vi "ConnectionHandler.vi"(6 "WebSocket Headers":variant, 8 "error in (no error)":errorcluster, 9 "Remote Address":string, 10 "connection ID":refnum<k5>, 11 "References In":variant) -> (0 "error out":errorcluster)   [LabVIEW 2013, in "Connection Handler.lvlib"]
uses:
  Connection Handler.lvlib
  ctl_ClientState.ctl
  <vilib>/Intelligent Energy/Message Queue Helper/ctl_QMH_Message_Typedef.ctl
  ctl_Message.ctl
  <vilib>/Intelligent Energy/Message Queue Helper/MessageQueueHelper.lvlib
  <vilib>/Intelligent Energy/WebSockets API/WebSockets/WebSockets.lvlib
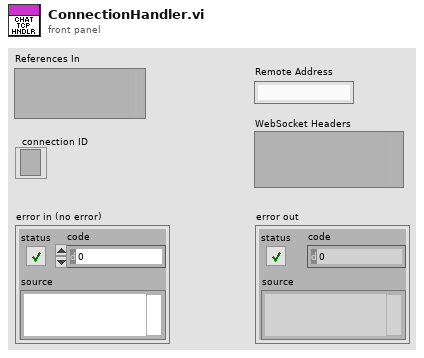
[diagram p1: front panel]
types:
  T1 = typedef "Connection Handler.lvlib/ctl_ClientState.ctl" = cluster{"Conn Ref":refnum<k5>, "IP Address":string, "Hostname":string, "User":cluster{"Username":string, "Read":bool, "Write":bool}}
  T2 = typedef "Connection Handler.lvlib/ctl_Message.ctl" = cluster{"username":string, "message":string}
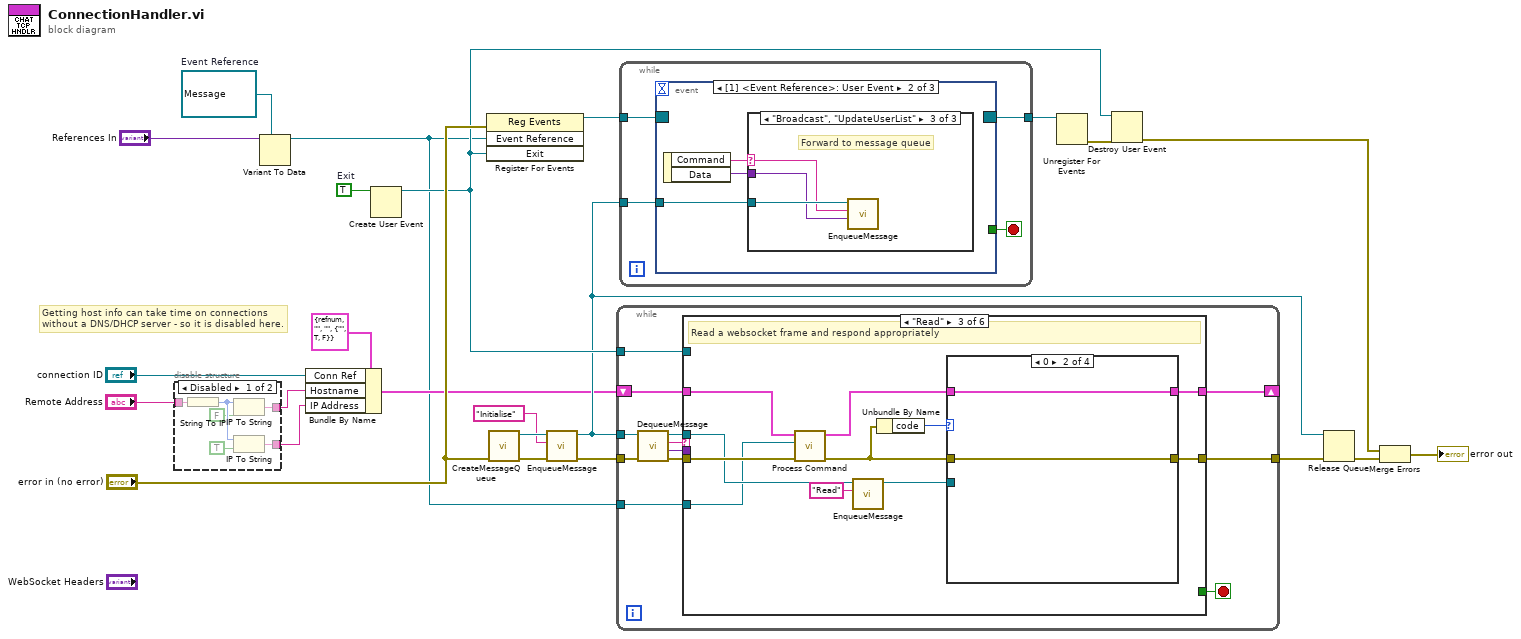
[diagram p0: block diagram]
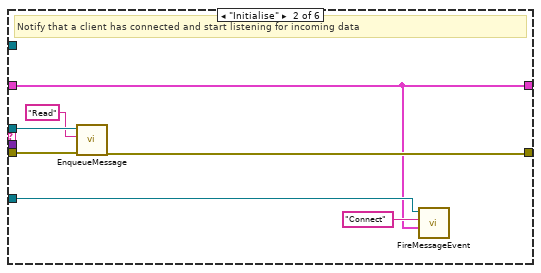
[diagram p4: hidden frame]
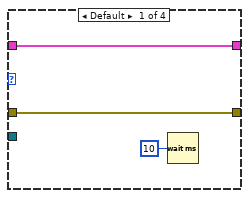
[diagram p5: hidden frame]
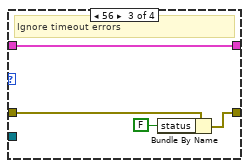
[diagram p6: hidden frame]
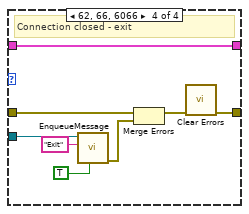
[diagram p7: hidden frame]
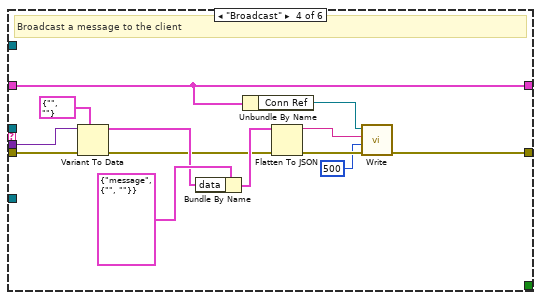
[diagram p8: hidden frame]
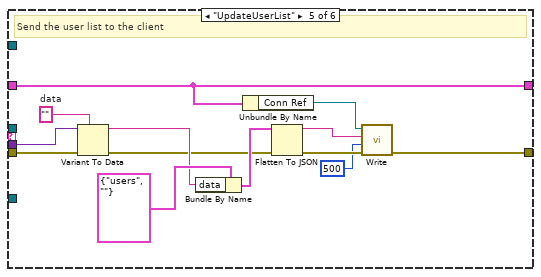
[diagram p9: hidden frame]
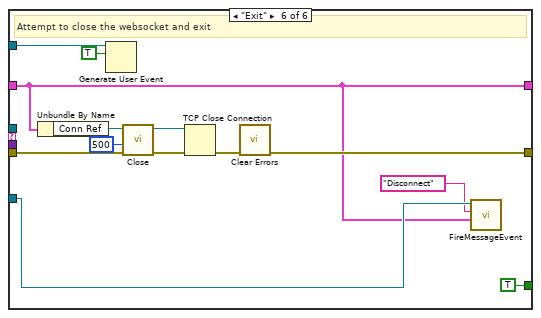
[diagram p10: hidden frame]
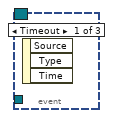
[diagram p11: hidden frame]
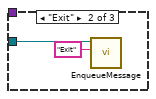
[diagram p13: hidden frame]
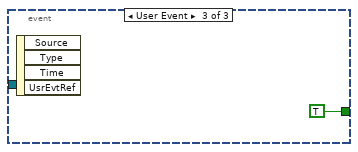
[diagram p14: hidden frame]
diagram:
  w2 = refnum<user-event> refnum  # Event Reference
  w18 = TRUE  # Exit
  # "Getting host info can take time on connections\nwithout a DNS/DHCP server - so it is disabled here."
  n1 = disable-structure shown="Disabled" {
    disable-tunnel: "Remote Address" -> [w27 w31]
    disable-tunnel: [w26 w31] -> w6
    disable-tunnel: [w25 w31] -> w5
    frame Disabled {
      n2 = String To IP(1:w27) -> (0:w30:u32)
      n3 = IP To String(1:FALSE ("dot notation? (F)"), 2:w30) -> (0:w25:string)
      n4 = IP To String(1:TRUE ("dot notation? (F)"), 2:w30) -> (0:w26:string)
    }
    frame Enabled {
    }
  }
  n5 = Variant To Data(type=w2, Variant="References In") -> (data=w1:refnum<user-event>)  [unwired: 1 in, 1 out]
  n6 = Bundle By Name(cluster=T1 {"Conn Ref"=refnum, "IP Address"="", "Hostname"="", "User"={"Username"="", "Read"=TRUE, "Write"=FALSE}} ("State out"), "Conn Ref"="connection ID", "Hostname"=w5, "IP Address"=w6) -> (w4:T1)
  n7 = Create User Event(user event datatype=w18) -> (user event=w15:refnum<user-event>)  [unwired: 1 in, 1 out]
  n8 = register-events(error in="error in (no error)", w1, w15) -> (reference out=w24:refnum<event-registration>)  [unwired: 1 in, 1 out]
  n9 = call <vilib>:"CreateMessageQueue.vi"("error in (no error)"="error in (no error)") -> ("error out"=w14:errorcluster, "queue out"=w11:refnum<queue>)  [unwired: 8 in, 1 out]
  n10 = call <vilib>:"EnqueueMessage.vi"("error in (no error)"=w14, "Message"="Initialise", "queue in"=w11) -> ("error out"=w13:errorcluster, "queue out"=w12:refnum<queue>)  [unwired: 7 in]
  n11 = while {
    tunnel: w12 -> [w43]
    tunnel: w13 -> [w42]
    tunnel: [w33] -> w22
    shift-right: [w36] -> _
    shift-left: w4 -> [w35]
    tunnel: w15 -> [w34]
    tunnel: w1 -> [w32]
    stop <- w37 stop-if-true
    n12 = call <vilib>:"DequeueMessage.vi"("error in (no error)"=w42, "queue in"=w43) -> ("error out"=w40:errorcluster, "Data"=w38:variant, "Command"=w41:string, "queue out"=w39:refnum<queue>)  [unwired: 6 in]
    n13 = case shown="\"Read\"" w41 {
      tunnel: w40 -> [w45 w52 w63 w90 w103 w115]
      tunnel: [w45 w49 w60 w92 w105 w110] -> w33
      tunnel: w39 -> [_ w51 w59 _ _ _]
      tunnel: w38 -> [_ _ _ w89 w102 _]
      tunnel: [_ _ _ _ _ TRUE] -> w37
      tunnel: [w44 w46 w56 w93 w106 w107] -> w36
      tunnel: w35 -> [w44 w46 w54 w93 w106 w107]
      tunnel: w34 -> [_ _ _ _ _ w117]
      tunnel: w32 -> [_ w47 w53 _ _ w109]
      frame Default {
      }
      frame "Initialise" {
        # "Notify that a client has connected and start listening for incoming data"
        n14 = call <vilib>:"EnqueueMessage.vi"("error in (no error)"=w52, "Message"="Read", "queue in"=w51) -> ("error out"=w49:errorcluster)  [unwired: 7 in, 1 out]
        n15 = call <vilib>:"FireMessageEvent.vi"("Data"=w46, "Command"="Connect", "User Event in"=w47) -> ()  [unwired: 7 in, 2 out]
      }
      frame "Read" {
        # "Read a websocket frame and respond appropriately"
        n16 = call "Process Command.vi"("error in (no error)"=w63, "user event in"=w53, "State in"=w54) -> ("error out"=w61:errorcluster, "State out"=w57:T1)  [unwired: 7 in]
        n17 = call <vilib>:"EnqueueMessage.vi"("Message"="Read", "queue in"=w59) -> ("queue out"=w55:refnum<queue>)  [unwired: 8 in, 1 out]
        n18 = Unbundle By Name(w61) -> ("code"=w62:i32)
        n19 = case shown="0" w62 {
          tunnel: w61 -> [w65 w68 w72 w76]
          tunnel: [w65 w68 w70 w74] -> w60
          tunnel: w57 -> [w64 w67 w69 w77]
          tunnel: [w64 w67 w69 w77] -> w56
          tunnel: w55 -> [_ _ _ w80]
          frame Default {
            n20 = Wait (ms)(milliseconds to wait=u32 10) -> ()  [unwired: 1 out]
          }
          frame 0 {
          }
          frame 56 {
            # "Ignore timeout errors"
            n21 = Bundle By Name(cluster=w72, "status"=FALSE) -> (w70:errorcluster)
          }
          frame 62, 66, 6066 {
            # "Connection closed - exit"
            n22 = call <vilib>:"EnqueueMessage.vi"("Priority?"=TRUE, "Message"="Exit", "queue in"=w80) -> ("error out"=w75:errorcluster)  [unwired: 7 in, 1 out]
            n23 = Merge Errors(w76, w75) -> (w73:errorcluster)
            n24 = call <vilib>:"Clear Errors.vi"("error in (no error)"=w73) -> ("error out"=w74:errorcluster)  [unwired: 6 in]
          }
        }
      }
      frame "Broadcast" {
        # "Broadcast a message to the client"
        n25 = Variant To Data(error in=w90, type=T2 {"username"="", "message"=""} ("data"), Variant=w89) -> (data=w86:T2, error out=w84:errorcluster)
        n26 = Bundle By Name(cluster=cluster{"command":string, "data":T2} {"command"="message", "data"={"username"="", "message"=""}}, "data"=w86) -> (w85:cluster{"command":string, "data":T2})
        n27 = Unbundle By Name(w93) -> ("Conn Ref"=w91:refnum<k5>)
        n28 = Flatten To JSON(anything=w85, error in (no error)=w84) -> (JSON string=w82:string, 11:w83:errorcluster)  [unwired: 1 in]
        n29 = call <vilib>:"Write.vi"("error in (no error)"=w83, "timeout ms (5000)"=500, "Data"=w82, "WebSocket Connection in"=w91) -> ("error out"=w92:errorcluster)  [unwired: 6 in, 1 out]
      }
      frame "UpdateUserList" {
        w94 = ""  # data
        # "Send the user list to the client"
        n30 = Variant To Data(error in=w103, type=w94, Variant=w102) -> (data=w100:string, error out=w98:errorcluster)
        n31 = Bundle By Name(cluster=cluster{"command":string, "data":string} {"command"="users", "data"=""}, "data"=w100) -> (w99:cluster{"command":string, "data":string})
        n32 = Unbundle By Name(w106) -> ("Conn Ref"=w104:refnum<k5>)
        n33 = Flatten To JSON(anything=w99, error in (no error)=w98) -> (JSON string=w96:string, 11:w97:errorcluster)  [unwired: 1 in]
        n34 = call <vilib>:"Write.vi"("error in (no error)"=w97, "timeout ms (5000)"=500, "Data"=w96, "WebSocket Connection in"=w104) -> ("error out"=w105:errorcluster)  [unwired: 6 in, 1 out]
      }
      frame "Exit" {
        # "Attempt to close the websocket and exit"
        n35 = Unbundle By Name(w107) -> ("Conn Ref"=w111:refnum<k5>)
        n36 = Generate User Event(user event=w117, event data cluster=TRUE ("event data")) -> ()  [unwired: 2 in, 2 out]
        n37 = call <vilib>:"Close.vi"("error in (no error)"=w115, "timeout ms (5000)"=500, "WebSocket Connection in"=w111) -> ("error out"=w114:errorcluster, "WebSocket Connection in"=w113:refnum<k5>)  [unwired: 7 in]
        n38 = TCP Close Connection(connection ID=w113, error in (no error)=w114) -> (error out=w118:errorcluster)  [unwired: 1 in, 1 out]
        n39 = call <vilib>:"Clear Errors.vi"("error in (no error)"=w118) -> ("error out"=w110:errorcluster)  [unwired: 6 in]
        n40 = call <vilib>:"FireMessageEvent.vi"("Data"=w107, "Command"="Disconnect", "User Event in"=w109) -> ()  [unwired: 7 in, 2 out]
      }
    }
  }
  n41 = while {
    tunnel: w24 -> [w123]
    tunnel: [w122] -> w23
    tunnel: w12 -> [w120]
    stop <- w121 stop-if-true
    n42 = event shown="[1] <Event Reference>: User Event" {
      selector: w123 -> [_ _ _]
      dyn-events: [_ _ _] -> w122
      timeout: _ -> [_ _ _]
      tunnel: [_ _ TRUE] -> w121
      tunnel: w120 -> [_ w126 _]
      event Timeout {
        n43 = event-data() -> ()  [unwired: 1 in, 3 out]
      }
      event User Event {
        n44 = event-data() -> ("Command"=w125:string, "Data"=w124:variant)  [unwired: 1 in]
        n45 = case shown="\"Broadcast\", \"UpdateUserList\"" w125 {
          selector: w125 -> [_ _ w130]
          tunnel: w126 -> [_ w128 w131]
          tunnel: w124 -> [_ _ w129]
          frame Default {
          }
          frame "Exit" {
            n46 = call <vilib>:"EnqueueMessage.vi"("Message"="Exit", "queue in"=w128) -> ()  [unwired: 8 in, 2 out]
          }
          frame "Broadcast", "UpdateUserList" {
            # "Forward to message queue"
            n47 = call <vilib>:"EnqueueMessage.vi"("Variant"=w129, "Message"=w130, "queue in"=w131) -> ()  [unwired: 7 in, 2 out]
          }
        }
      }
      event User Event {
        n48 = event-data() -> ()  [unwired: 1 in, 4 out]
      }
    }
  }
  n49 = Unregister For Events(event registration refnum=w23) -> (error out=w17:errorcluster)  [unwired: 1 in]
  n50 = Destroy User Event(user event=w15, error in=w17) -> (error out=w16:errorcluster)
  n51 = Release Queue(queue=w12, error in (no error)=w22) -> (error out=w21:errorcluster)  [unwired: 1 in, 2 out]
  n52 = Merge Errors(w16, w21) -> (→"error out":errorcluster)
